vi "Stepper shift to Force3.vi"(4 "F1/L1/F0/F2/L2":dbl[](array[numeric]), 7 "Stepper Shift":dbl[](array[numeric])) -> (0 "Fmax/decay/Fmin":dbl[](array[numeric]), 3 "Force(pN)":dbl[](array[numeric]))   [LabVIEW 2018]
panel:
  out "XY Graph":cluster{"Y":dbl[], "Y":dbl[]}[](graph)
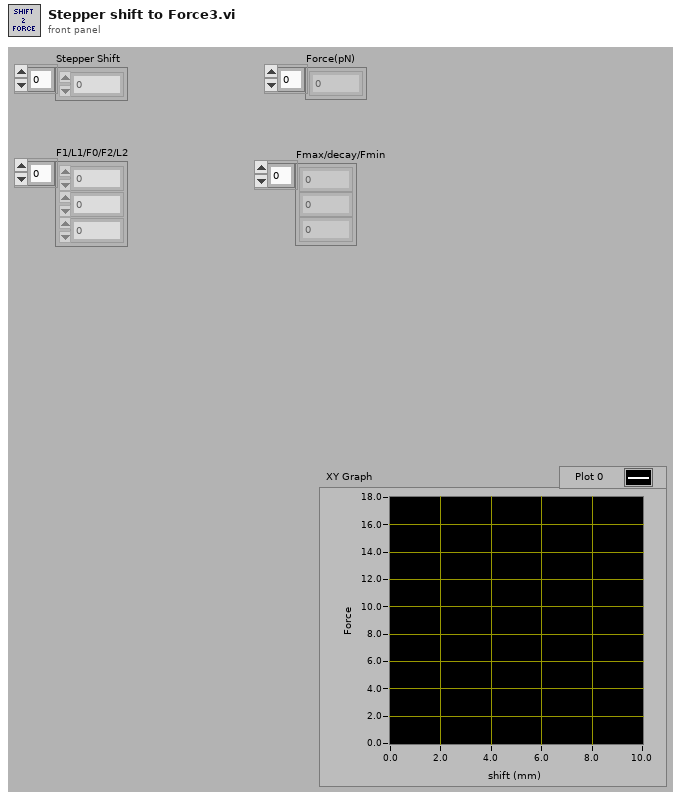
[diagram p1: front panel]
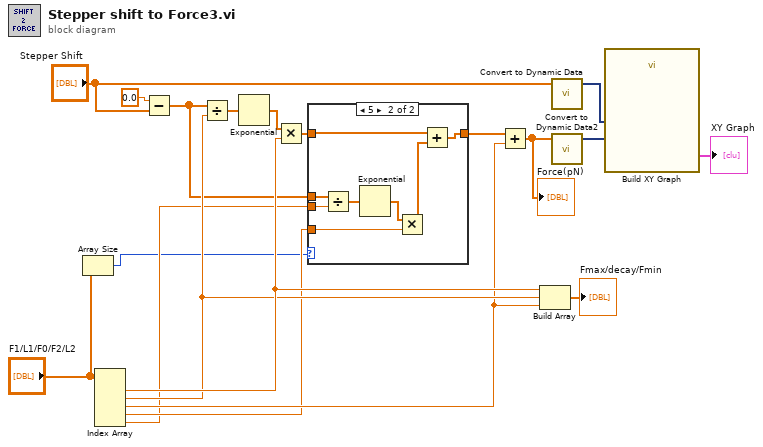
[diagram p0: block diagram]
diagram:
  n1 = Array Size(array="F1/L1/F0/F2/L2") -> (size(s)=w3:i32)
  n2 = Index Array(array="F1/L1/F0/F2/L2") -> (element #1=w10:dbl, element #2=w9:dbl, element #3=w8:dbl, element #4=w6:dbl, element #5=w5:dbl)  [unwired: 5 in]
  n3 = Subtract(x=0.0, y="Stepper Shift") -> (x-y=w7:dbl[])
  n4 = Divide(x=w7, y=w9) -> (x/y=w18:dbl[])
  n5 = Exponential(1:w18) -> (0:w17:dbl[])
  n6 = Multiply(x=w17, y=w10) -> (x*y=w1:dbl[])
  n7 = case shown="5" w3 {
    tunnel: w7 -> [_ w26]
    tunnel: w6 -> [_ w25]
    tunnel: w5 -> [_ w24]
    tunnel: [w20 w21] -> w2
    tunnel: w1 -> [w20 w23]
    frame 0, Default {
    }
    frame 5 {
      n8 = Divide(x=w26, y=w24) -> (x/y=w27:dbl[])
      n9 = Exponential(1:w27) -> (0:w28:dbl[])
      n10 = Multiply(x=w28, y=w25) -> (x*y=w22:dbl[])
      n11 = Add(x=w23, y=w22) -> (x+y=w21:dbl[])
    }
  }
  n12 = Add(x=w2, y=w8) -> (x+y=w12:dbl[])
  "Force(pN)" <- w12
  n13 = Build Array(w10, w9, w8) -> (→"Fmax/decay/Fmin":dbl[])
  n14 = call "Convert to Dynamic Data"("Array"="Stepper Shift") -> ("Dynamic Data Type"=w14:dynamicdata)  [unwired: 3 in]
  n15 = call "Convert to Dynamic Data2"("Array"=w12) -> ("Dynamic Data Type"=w13:dynamicdata)  [unwired: 3 in]
  n16 = call "Build XY Graph"("Y Input"=w13, "X Input"=w14) -> ("XY Graph"=→"XY Graph":cluster{"Y":dbl[], "Y":dbl[]}[])  [unwired: 3 in, 6 out]
